vi "Static Read.vi"(8 "error in (no error)":errorcluster, 11 "Abs_U8 Integer in":refnum<class "Abs_U8 Integer.lvclass">) -> (0 "error out":errorcluster, 2 "Value":u8, 3 "Abs_U8 Integer out":refnum<class "Abs_U8 Integer.lvclass">)   [LabVIEW 2021, in "Abs_U8 Integer.lvclass"]
uses:
  Abs_U8 Integer.lvclass
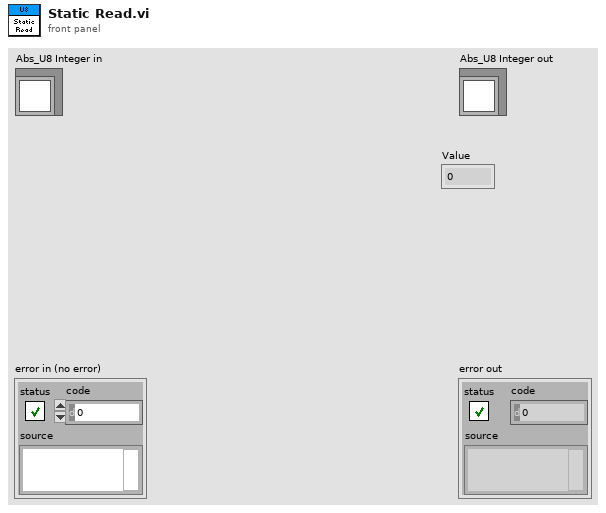
[diagram p1: front panel]
types:
  T1 = typedef "Abs_U8 Integer.lvclass/Type.ctl" = u8
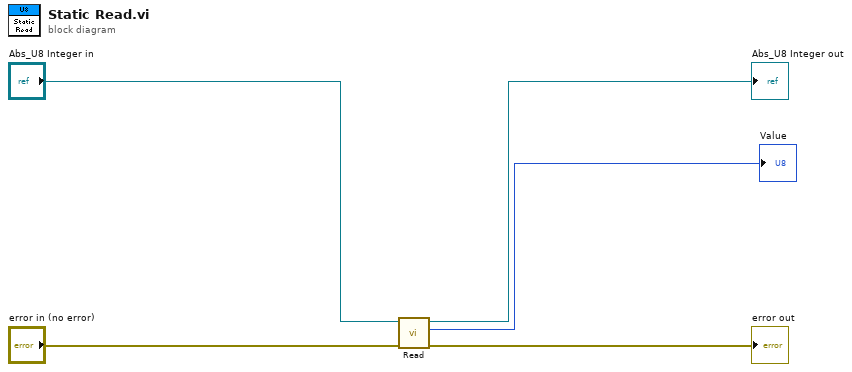
[diagram p0: block diagram]
diagram:
  n1 = call-dynamic "Read.vi"("error in (no error)"="error in (no error)", "Double Float.lvclass_340760 in"="Abs_U8 Integer in") -> ("error out"=→"error out":errorcluster, "Value"=→"Value":T1, "Double Float.lvclass_340760 out"=→"Abs_U8 Integer out":refnum<class "Abs_U8 Integer.lvclass">)  [unwired: 7 in]
